vi "ep_Digital Data to U16 (1 Sample).vi"(8 "error in":errorcluster, 11 "digital signal":bool[](array[boolean])) -> (0 "error out":errorcluster, 3 "U16 digital data":u16[](array[numeric]))   [LabVIEW 2011, in "NI_EP_COMTRADE.lvlib"]
uses:
  <vilib>/addons/Electrical Power/File IO/NI_EP_COMTRADE.lvlib
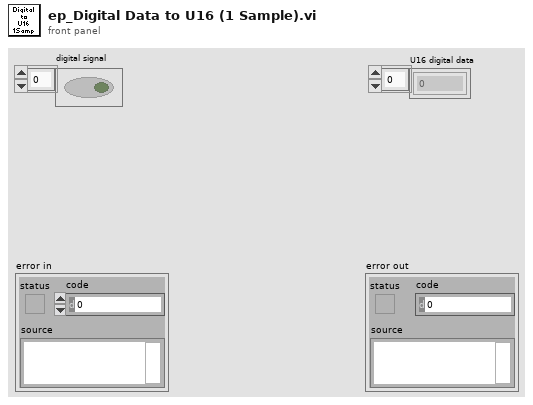
[diagram p1: front panel]
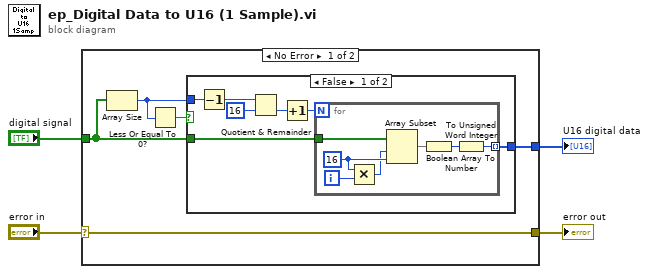
[diagram p0: block diagram]
diagram:
  n1 = case shown="No Error" "error in" {
    selector: "error in" -> [w9 w24]
    tunnel: "digital signal" -> [w6 _]
    tunnel: [w9 w24] -> w2
    tunnel: [w5 _] -> w1
    frame No Error {
      n2 = Array Size(array=w6) -> (size(s)=w7:i32)
      n3 = Less Or Equal To 0?(x=w7) -> (x <= 0?=w8:bool)
      n4 = case shown="False" w8 {
        tunnel: w7 -> [w13 _]
        tunnel: w6 -> [w11 _]
        tunnel: [w10 _] -> w5
        frame False {
          n5 = Decrement(x=w13) -> (x-1=w14:i32)
          n6 = Quotient & Remainder(x=w14, y=16) -> (floor(x/y)=w15:i32)  [unwired: 1 out]
          n7 = Increment(x=w15) -> (x+1=w12:i32)
          n8 = for {
            N: w12 -> [_]
            tunnel: w11 -> [w23]
            tunnel: [w17] -> w10 mode=indexing
            i -> [w20]
            w22 = 16 ("x")
            n9 = Multiply(x=w22, y=w20) -> (x*y=w21:i32)
            n10 = Array Subset(array=w23, index=w21, length=w22) -> (w19:bool[])
            n11 = Boolean Array To Number(Boolean array=w19) -> (number=w18:u32)
            n12 = To Unsigned Word Integer(number=w18) -> (unsigned 16bit integer=w17:u16)
          }
        }
        frame True {
        }
      }
    }
    frame Error {
    }
  }
  "error out" <- w2
  "U16 digital data" <- w1
